vi "运维调试_总磷总氮.vi"() -> ()   [LabVIEW 2016, in "斯坦道仪器.lvlib"]
uses:
  <vilib>/Platform/TimedLoop/XDataNode/timing_clust.ctl
  <vilib>/Platform/TimedLoop/XDataNode/nitl_modes.ctl
  <vilib>/Platform/TimedLoop/XDataNode/wakeup.ctl
  <vilib>/Utility/miscctls.llb/LVPointTypeDef.ctl
  <vilib>/Utility/config.llb/Read Key (Double).vi
  <vilib>/Utility/config.llb/Write Key (Double).vi
  <vilib>/Platform/TimedLoop/XDataNode/XDataNode.xnode
  <vilib>/Platform/TimedLoop/XDataNode/XDNodeRunTimeDep.lvlib
  <vilib>/Utility/config.llb/NI_LVConfig.lvlib
panel:
  out "字符串":string
  out "总氮稀释倍数":dbl
  out "固件版本号":string
  in  "数组":string[](array[string])
  in  "备用系数写入":bool
  in  "备用系数读取":bool
  in  "备用系数":T1
  in  "量程切换阈值写入":bool
  in  "量程切换阈值读取":bool
  in  "量程切换阈值":cluster{"阈值":dbl, "标液浓度":dbl}
  in  "参数下拉列表":enum16{"总磷", "总氮"}(ring)
  in  "量程下拉列表":enum16{"低量程", "高量程"}(ring)
  in  "测量模式下拉列表":enum16{"水样测量", "空白核查", "跨度核查", "标样核查", "加标回收"}(ring)
  in  "公式":cluster{"X^2":dbl, "X":dbl, "b":dbl}
  in  "写公式":bool
  in  "读公式":bool
  in  "精度":dbl=4.0
  in  "样品5 F0":dbl
  in  "样品5 F1":dbl
  in  "样品4 F1":dbl
  in  "样品4 F0":dbl
  in  "样品3 F0":dbl
  in  "样品3 F1":dbl
  in  "样品2 F0":dbl
  in  "样品2 F1":dbl
  in  "样品1 F1":dbl
  in  "样品1 F0":dbl
  in  "method":u16(ring) items=["最小二乘", "最小绝对残差", "Bisquare"]
  in  "模型":enum32{"线性", "多项式"}(ring)
  out "r^2":dbl format="%.7g"
  out "拟合公式":string
  in  "样品2启用":bool
  in  "样品5启用":bool
  in  "样品4启用":bool
  in  "样品3启用":bool
  in  "样品1启用":bool
  in  "标液浓度5":dbl
  out "测量吸光度5":dbl
  in  "标液浓度4":dbl
  out "测量吸光度4":dbl
  in  "标液浓度3":dbl
  out "测量吸光度3":dbl
  in  "标液浓度2":dbl
  out "测量吸光度2":dbl
  out "测量吸光度1":dbl
  in  "标液浓度1":dbl
  out "XY图":cluster{"X Values":dbl[], "Y Values":dbl[]}[](graph)
  in  "返回":bool
  in  "设置":bool
  out "序列号":string="序列号"
  out "总氮测量数据":T2(xcontrol)
  out "总磷测量数据":T2(xcontrol)
  out "集成报警信息":string
  out "设置值":dbl
  out "定时启动":bool
  out "总磷总氮运行状态":T3(xcontrol)
  in  "停止":bool
  in  "手动启动":bool
  in  "单步测试":bool
  in  "总磷氨氮调试":u16[](xcontrol)
  out "F3":sgl format="%#.6f"
  out "F2":sgl format="%#.6f"
  out "F1":sgl format="%#.6f"
  out "F0":sgl format="%#.6f"
  out "多列列表框":i32(listbox)
  # "COM5"
  # "参数设置"
  # "标液浓度"
  # "F0"
  # "F1"
  # "吸光值显示"
  # "样品一"
  # "辅\n助\n计\n算\n区"
  # "样品二"
  # "样品三"
  # "样品四"
  # "样品五"
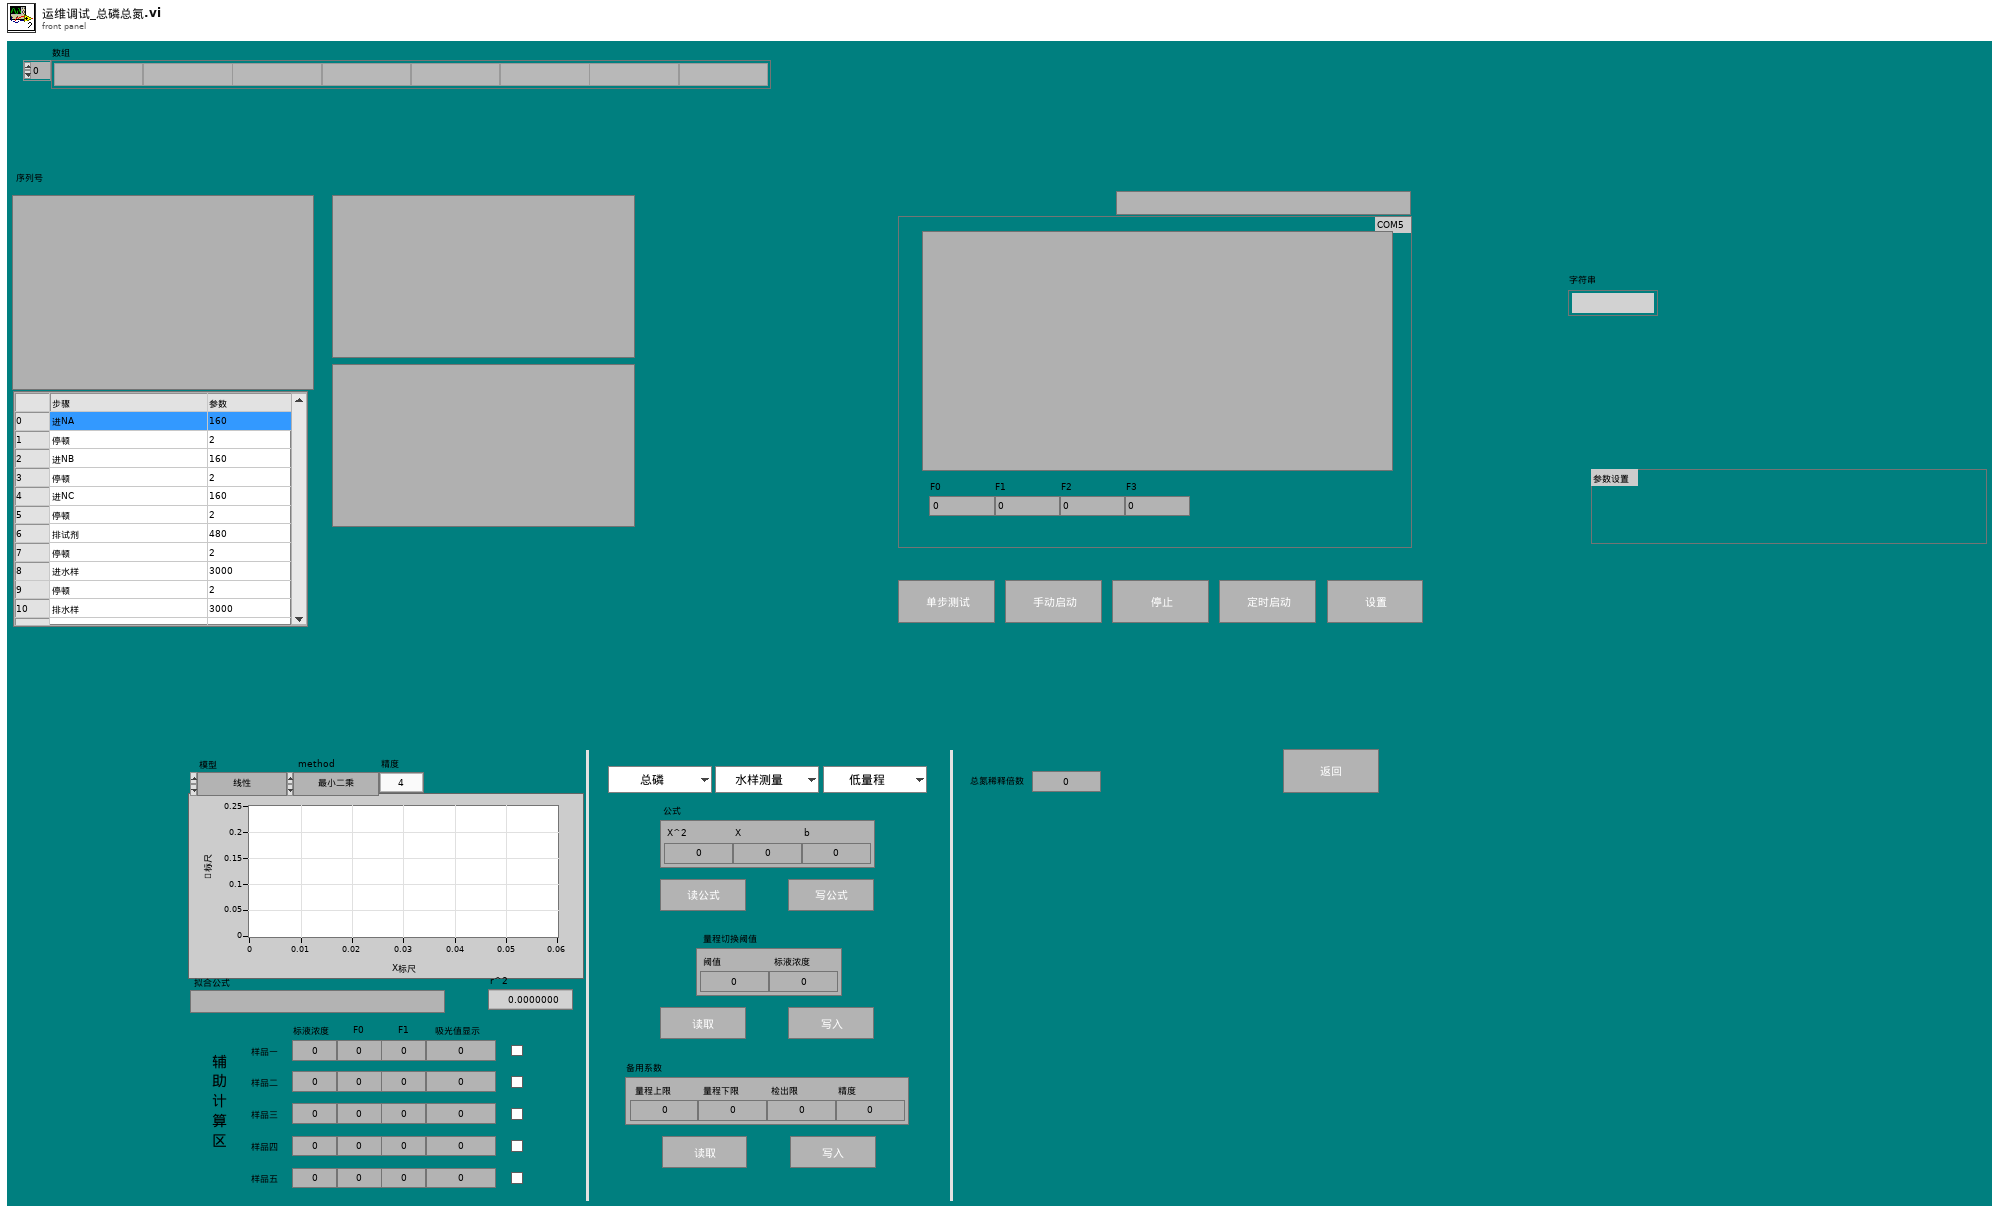
[diagram p1: front panel]
types:
  T1 = cluster{"量程上限":dbl, "量程下限":dbl, "检出限":dbl, "精度":dbl}
  T2 = cluster{"flowid":u16, "测量精度":u16, "测量数据区":cluster{"因子编码":u32, "单位":u16, "标样参考值":sgl, "水样数据时间":timestamp, "水样实测值":sgl, "水样数据标识":string, "标样数据时间":timestamp, "标样实测值":sgl, "标样数据标识":string, "空白数据时间":timestamp, "空白实测值":sgl, "空白数据标识":string, "零点核查数据时间":timestamp, "零点核查实测值":sgl, "零点核查数据标识":string, "跨度核查数据时间":timestamp, "跨度核查实测值":sgl, "跨度核查数据标识":string, "加标回收数据时间":timestamp, "加标回收实测值":sgl, "加标回收数据标识":string, "平行样数据时间":timestamp, "平行样实测值":sgl, "平行样数据标识":string, "F0":sgl, "F1":sgl, "F2":sgl, "F3":sgl, "F4":sgl, "F5":sgl, "F6":sgl, "F7":sgl, "温度":sgl, "湿度":sgl, "X值":sgl}}
  T3 = cluster{"系统时间":timestamp, "工作状态":enum16{"空闲", "水样测试", "标样核查", "零点核查", "跨度核查", "空白测试", "平行样测试", "加标回收", "空白校准", "标样校准", "初始化（清洗）"}, "测量模式":enum16{"待机", "连续模式", "周期模式", "定点模式", "受控模式", "手动模式"}, "告警代码":enum16{"无告警", "缺试剂告警", "缺水样告警", "缺蒸馏水告警", "缺标液告警", "仪表漏液告警", "标定异常告警", "超量程告警", "加热异常", "低试剂预警", "超上限告警", "超下限告警", "仪表内部其他异常", "滴定异常告警", "电极异常告警", "量程切换告警", "参数设置告警", "PH电极电位异常", "电导率电极异常", "浊度光度异常", "溶解氧电极异常", "溶解氧光强异常", "温度异常告警", "PH异常告警", "溶解氧异常告警", "电导率异常告警", "浊度异常告警", "叶绿素异常告警", "藻密度异常告警", "蓝绿藻异常告警", "ORP异常告警", "氨氮异常告警", "清洁刷异常告警", "SD卡异常告警", "蓝牙异常告警", "Wifi异常告警", "流程异常告警"}, "故障代码":enum16{"无故障", "电机故障", "温度故障", "通讯故障", "滴定故障"}, "日志代码":u16, "软件版本":u16, "F0":sgl, "F1":sgl, "F2":sgl, "F3":sgl, "T":sgl, "H":sgl, "id":u16, "flowid":u16, "量程":u16}
  T4 = enum16{"待机", "启动氨氮", "氨氮测量中", "启动总磷", "总磷测量中", "延时"}
  T5 = typedef "LVPointTypeDef.ctl" = cluster{"Horizontal":i16, "Vertical":i16}
  T6 = cluster{"因子编码":u32, "单位":u16, "标样参考值":sgl, "水样数据时间":timestamp, "水样实测值":sgl, "水样数据标识":string, "标样数据时间":timestamp, "标样实测值":sgl, "标样数据标识":string, "空白数据时间":timestamp, "空白实测值":sgl, "空白数据标识":string, "零点核查数据时间":timestamp, "零点核查实测值":sgl, "零点核查数据标识":string, "跨度核查数据时间":timestamp, "跨度核查实测值":sgl, "跨度核查数据标识":string, "加标回收数据时间":timestamp, "加标回收实测值":sgl, "加标回收数据标识":string, "平行样数据时间":timestamp, "平行样实测值":sgl, "平行样数据标识":string, "F0":sgl, "F1":sgl, "F2":sgl, "F3":sgl, "F4":sgl, "F5":sgl, "F6":sgl, "F7":sgl, "温度":sgl, "湿度":sgl, "X值":sgl}
  T7 = enum16{"空闲", "水样测试", "标样核查", "零点核查", "跨度核查", "空白测试", "平行样测试", "加标回收", "空白校准", "标样校准", "初始化（清洗）"}
  T8 = typedef "XDNodeRunTimeDep.lvlib/timing_clust.ctl" = cluster{"Expected End [f-1]":u64, "Actual End [f-1]":u64, "Finished Late? [f-1]":bool, "Expected End [i-1]":u64, "Actual End [i-1]":u64, "Finished Late? [i-1]":bool, "Expected Start [i]":u64, "Actual Start [i]":u64, "Expected Start [f]":u64, "Actual Start [f]":u64, "Source Name":string, "Structure Name":string, "Period":i64, "Deadline":i64, "Offset":i64, "Start":i64, "Priority":i32, "Timeout":i32, "Mode":T9, "Wakeup Reason":T10, "Error":errorcluster, "Source Type":string, "Secondary Source Type":string, "Global End Time":u64, "Global Start Time":u64, "Frame Duration":u64, "Iteration Duration":u64, "Assigned CPU":i32, "I/O Scan Engine Mode":u32}
  T9 = typedef "XDNodeRunTimeDep.lvlib/nitl_modes.ctl" = enum32{"No Change", "Process missed periods, maintain original phase", "Discard missed periods, maintain original phase", "Process missed periods, ignore original phase", "Discard missed periods, ignore original phase"}
  T10 = typedef "XDNodeRunTimeDep.lvlib/wakeup.ctl" = enum32{"Normal", "Aborted", "Asynchronous wakeup", "Timing source error", "Timed loop error", "Timeout"}
  T11 = cluster{"启动模式":enum16{"标液测量", "水样测量", "零液测量", "盲样测量", "加标回收"}, "启动参数":u16, "量程":enum16{"低量程", "高量程"}}
  T12 = cluster{"时间标识":timestamp, "设备":string, "日志信息":string, "流程参数":string}
  T13 = cluster{"时间标识":timestamp, "设备":string, "日志信息":string}
  T14 = enum16{"无告警", "缺试剂告警", "缺水样告警", "缺蒸馏水告警", "缺标液告警", "仪表漏液告警", "标定异常告警", "超量程告警", "加热异常", "低试剂预警", "超上限告警", "超下限告警", "仪表内部其他异常", "滴定异常告警", "电极异常告警", "量程切换告警", "参数设置告警", "PH电极电位异常", "电导率电极异常", "浊度光度异常", "溶解氧电极异常", "溶解氧光强异常", "温度异常告警", "PH异常告警", "溶解氧异常告警", "电导率异常告警", "浊度异常告警", "叶绿素异常告警", "藻密度异常告警", "蓝绿藻异常告警", "ORP异常告警", "氨氮异常告警", "清洁刷异常告警", "SD卡异常告警", "蓝牙异常告警", "Wifi异常告警", "流程异常告警"}
  T15 = typedef "LVRowAndColumnUnsignedTypeDef.ctl" = cluster{"Row":u32, "Column":u32}
  T16 = typedef "NI_LVConfig.lvlib/Config Data RefNum.ctl" = refnum<k1>
  T17 = cluster{"站号":u16, "量程切换":enum32{"H", "L", "AUTO"}, "控制命令":enum16{"启动测量", "标样核查", "零点核查", "跨度核查", "空白测试", "平行样测试", "加标回收", "空白校准", "标样校准", "初始化（清洗）", "停止测试", "仪器重启", "校时", "模式设置", "测量间隔设置", "盲样测试"}, "模式设置":enum16{"待机", "连续模式", "周期模式", "定点模式", "受控模式", "手动模式"}, "测量间隔":u16}
  T18 = cluster{"站号":u16, "量程切换":enum32{"H", "L", "AUTO"}, "控制命令":enum16{"启动测量", "标样核查", "零点核查", "跨度核查", "空白测试", "平行样测试", "加标回收", "空白校准", "标样校准", "初始化（清洗）", "停止测试", "仪器重启", "校时", "模式设置", "测量间隔设置"}, "模式设置":enum16{"待机", "连续模式", "周期模式", "定点模式", "受控模式", "手动模式"}, "测量间隔":u16}
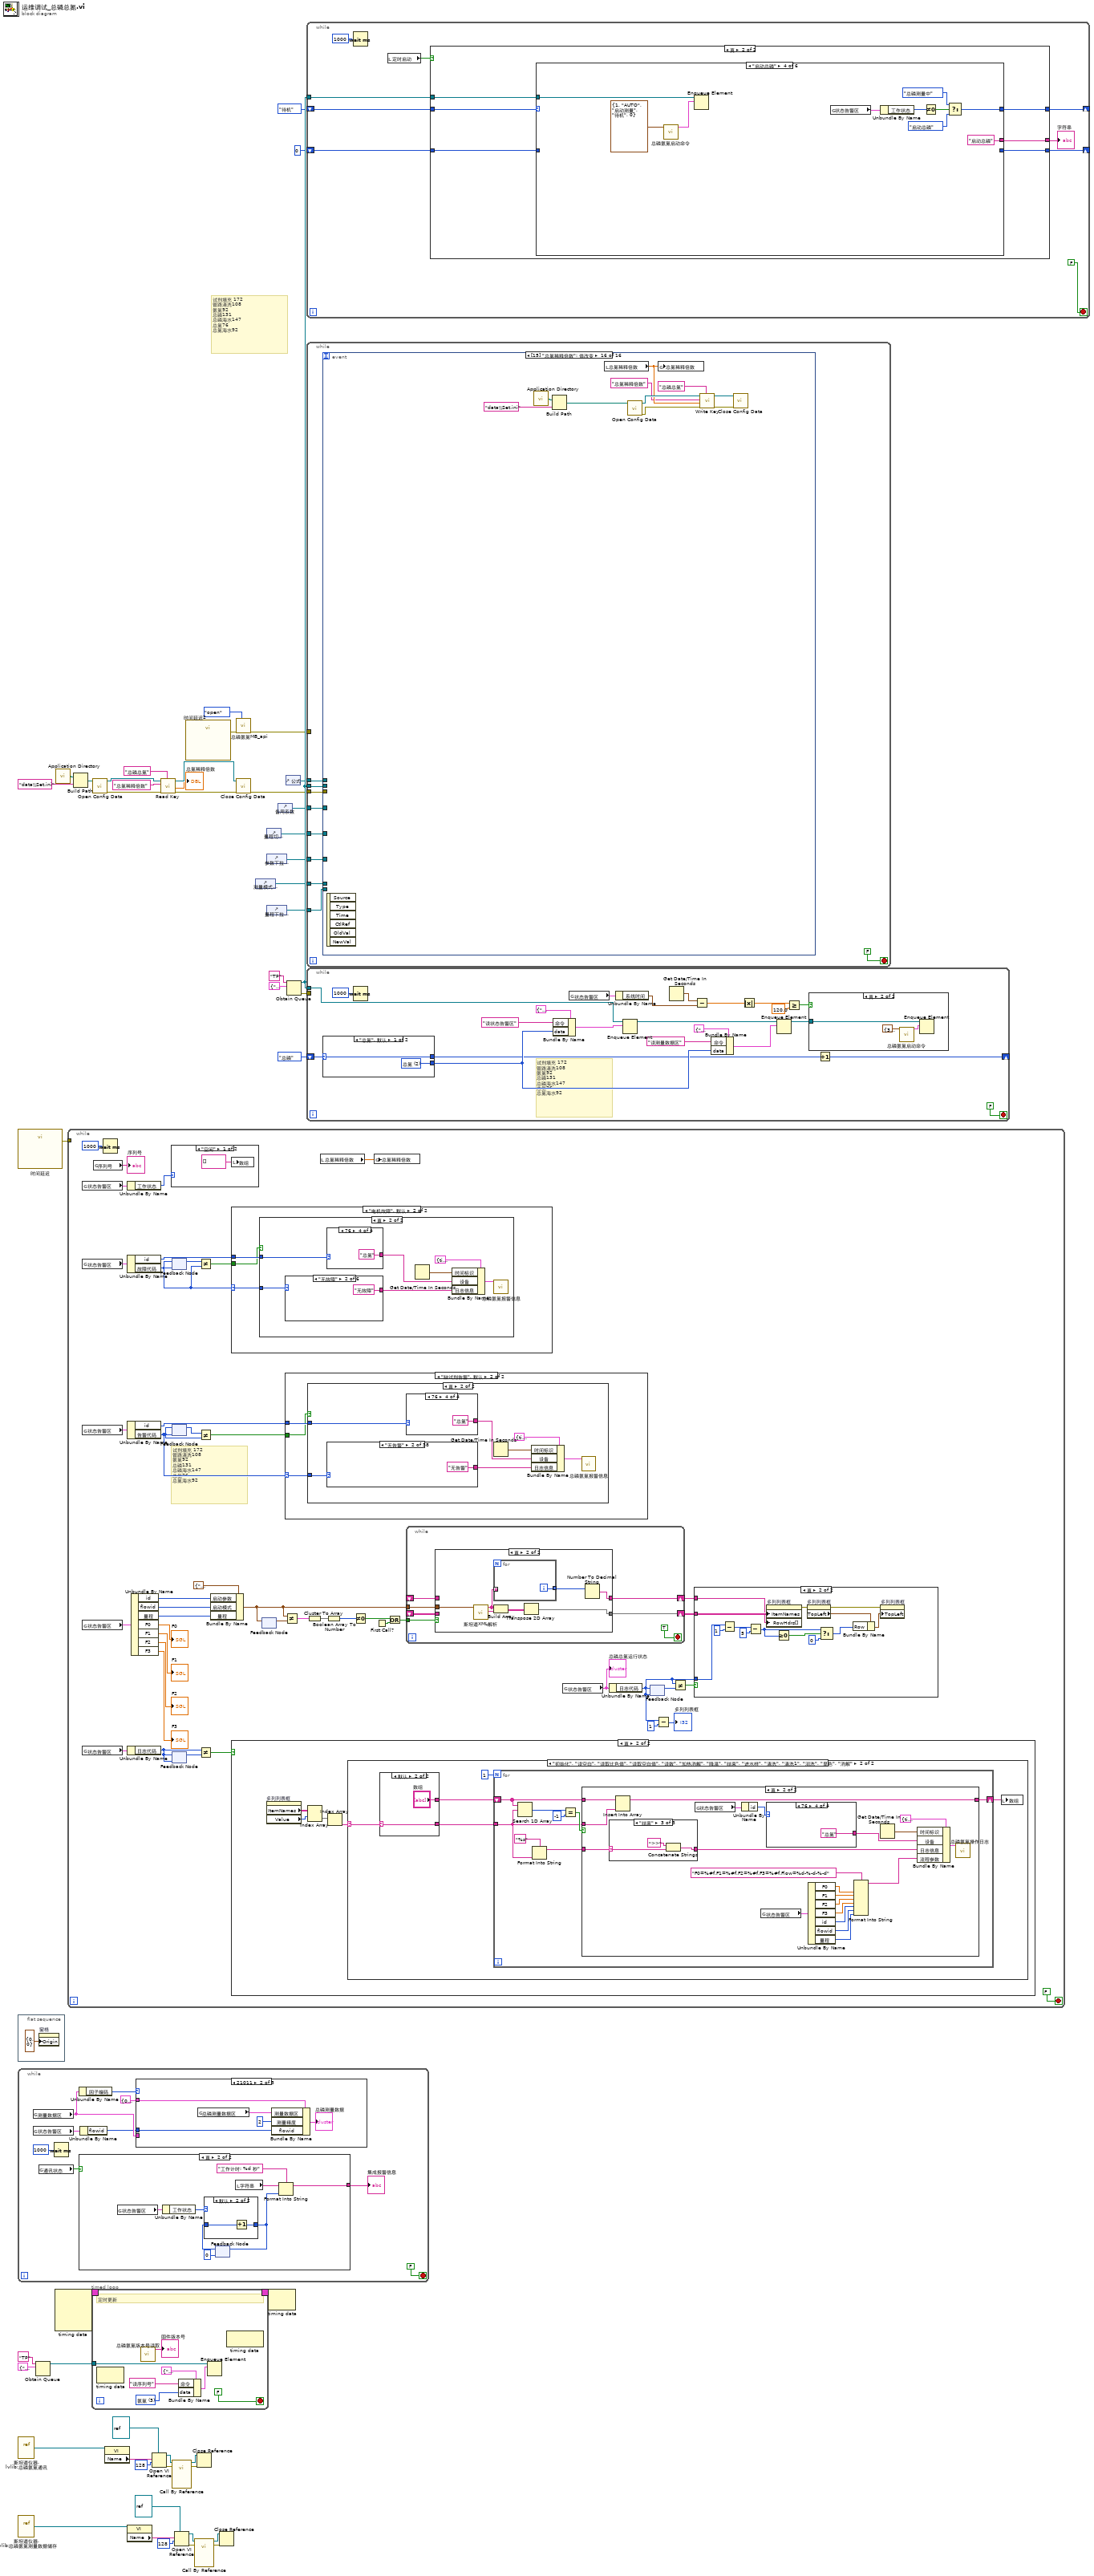
[diagram p0: block diagram]
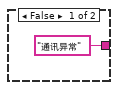
[diagram p2: hidden frame]
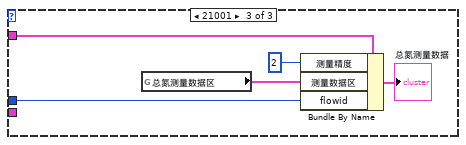
[diagram p5: hidden frame]
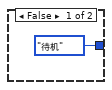
[diagram p6: hidden frame]
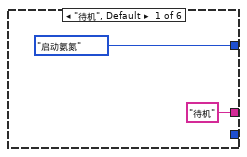
[diagram p7: hidden frame]
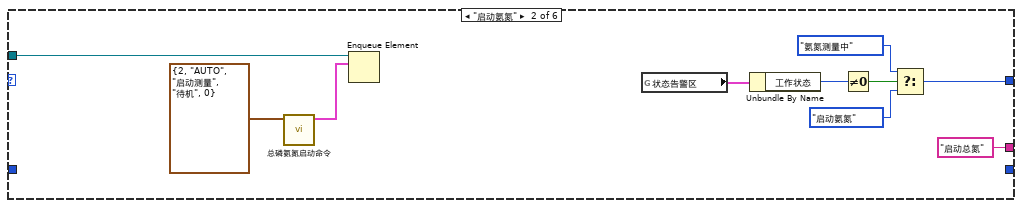
[diagram p8: hidden frame]
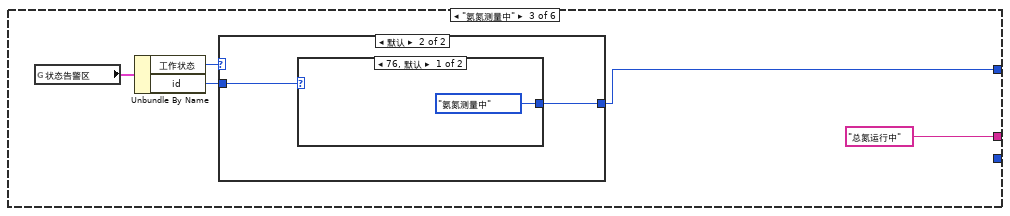
[diagram p9: hidden frame]
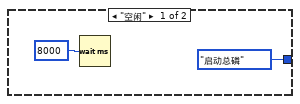
[diagram p10: hidden frame]
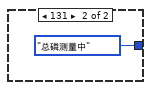
[diagram p11: hidden frame]
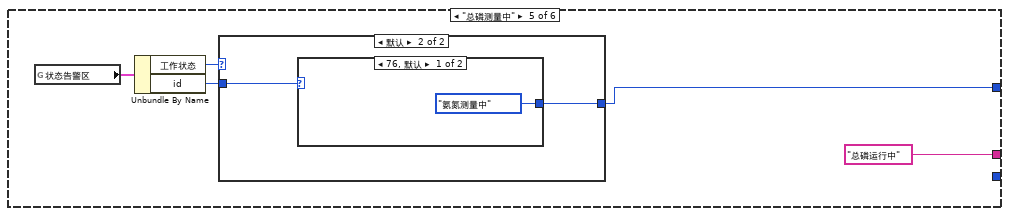
[diagram p12: hidden frame]
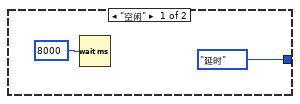
[diagram p13: hidden frame]
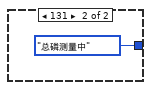
[diagram p14: hidden frame]
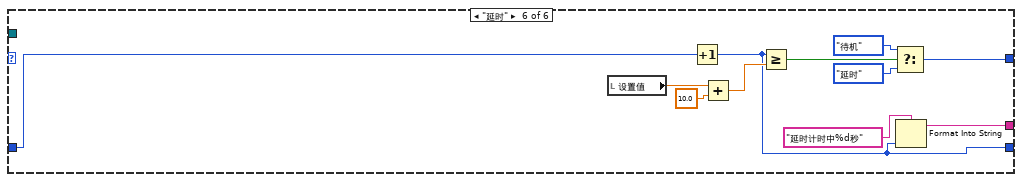
[diagram p15: hidden frame]
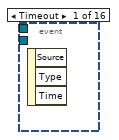
[diagram p16: hidden frame]
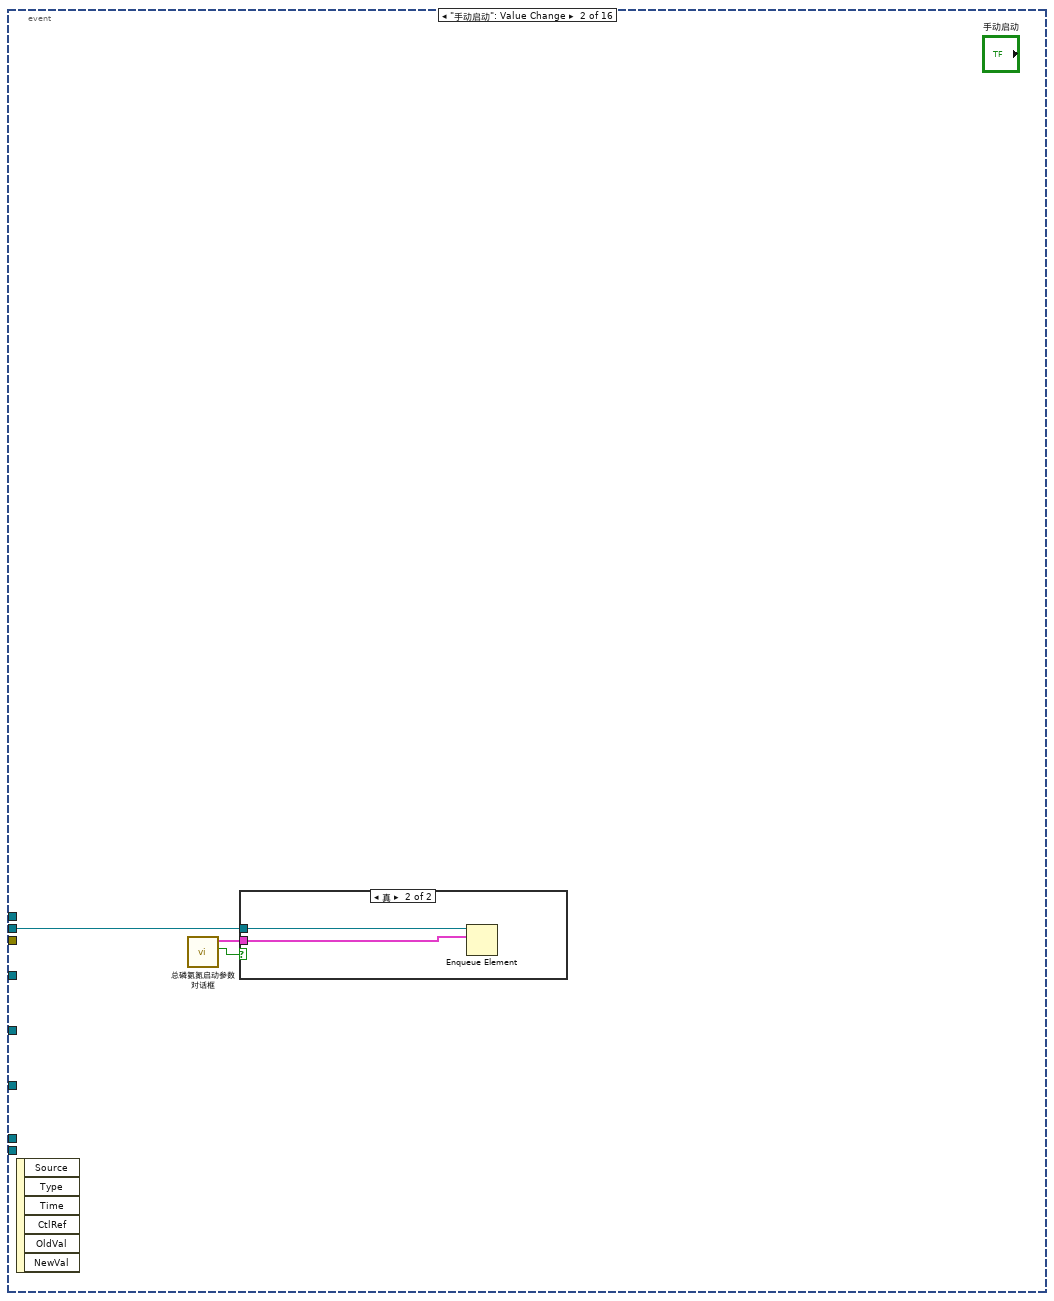
[diagram p17: hidden frame]
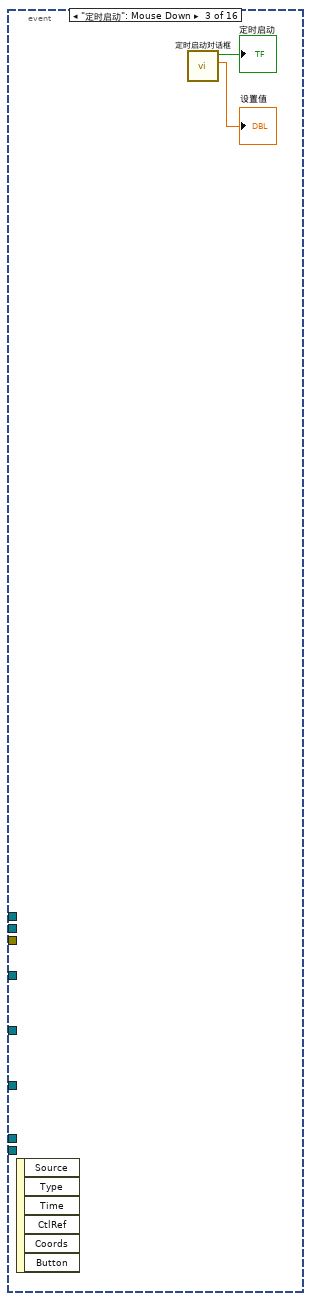
[diagram p19: hidden frame]
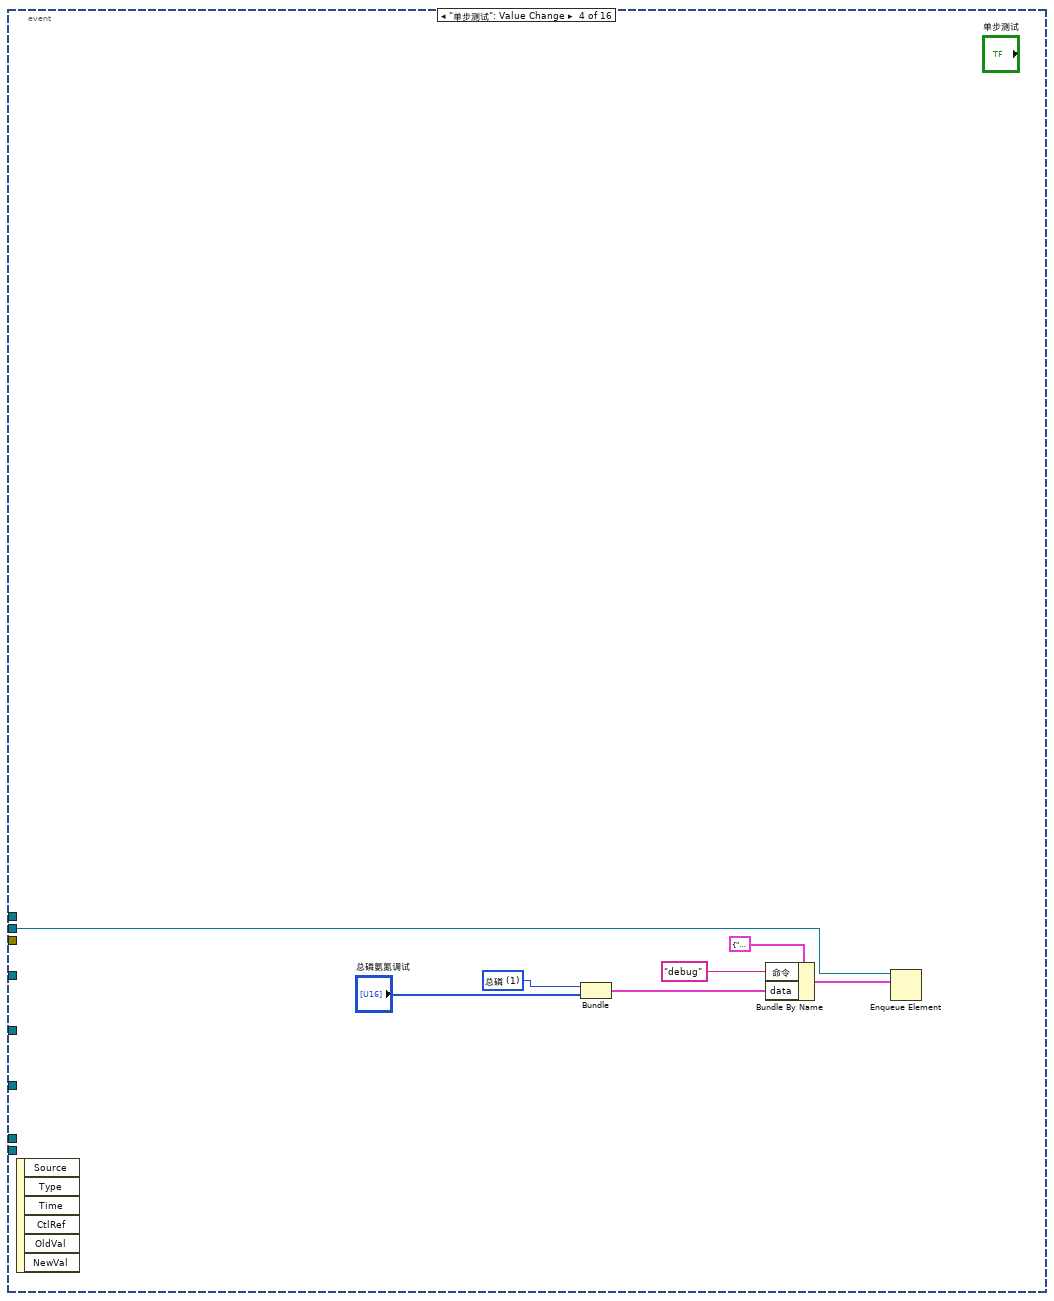
[diagram p20: hidden frame]
diagram:
  # "试剂填充 172 \n管路清洗108\n氨氮92\n总磷131\n总磷海水147\n总氮76\n总氮海水92"
  n1 = call "时间延迟"() -> ("error out"=w20:errorcluster)  [unwired: 11 in]
  n2 = flat-sequence {
    frame #0 {
      n3 = property on="窗格" class="Pane"("Origin"=T5 {"Horizontal"=0, "Vertical"=0} ("原点")) -> ()  [unwired: 2 in, 2 out]
    }
  }
  n4 = while {
    stop <- FALSE stop-if-true
    n5 = global read "VAR总磷氨氮全局变量.vi" "测量数据区"() -> (w57:T6)
    n6 = global read "VAR总磷氨氮全局变量.vi" "状态告警区"() -> (w53:T3)
    n7 = global read "VAR总磷氨氮全局变量.vi" "通讯状态"() -> (w55:bool)
    n8 = Wait (ms)(milliseconds to wait=u32 1000 ("等待时间（毫秒）")) -> ()  [unwired: 1 out]
    n9 = Unbundle By Name(w57) -> ("因子编码"=w56:u32)
    n10 = case shown="真" w55 {
      tunnel: ["通讯异常" ("集成报警信息") w62] -> w54
      frame False {
      }
      frame True {
        n11 = global read "VAR总磷氨氮全局变量.vi" "状态告警区"() -> (w68:T3)
        n12 = Unbundle By Name(w68) -> ("工作状态"=w67:T7)
        n13 = feedback #1(0) -> (w65:i32)
        n14 = case shown="默认" w67 {
          tunnel: w65 -> [_ w70]
          tunnel: [_ w69] -> w63
          frame "空闲" {
          }
          frame Default {
            n15 = Increment(x=w70) -> (x+1=w69:i32)
          }
        }
        n16 = feedback-in #1(w63) -> ()
        n17 = local read "字符串"() -> (w61:string)
        n18 = Format Into String(format string="工作计时: %d 秒" ("格式字符串"), initial string=w61, w63) -> (resulting string=w62:string)  [unwired: 1 in, 1 out]
      }
    }
    "集成报警信息" <- w54
    n19 = Unbundle By Name(w53) -> ("flowid"=w52:u16)
    n20 = case shown="21011" w56 {
      tunnel: w57 -> [_ _ _]
      tunnel: w52 -> [_ w73 w79]
      tunnel: T2 {"flowid"=0, "测量精度"=0, "测量数据区"={"因子编码"=0, "单位"=0, "标样参考值"=0.0, "水样数据时间"=timestamp(0 s since 1904-01-01), "水样实测值"=0.0, "水样数据标识"="", "标样数据时间"=timestamp(0 s since 1904-01-01), "标样实测值"=0.0, "标样数据标识"="", "空白数据时间"=timestamp(0 s since 1904-01-01), "空白实测值"=0.0, "空白数据标识"="", "零点核查数据时间"=timestamp(0 s since 1904-01-01), "零点核查实测值"=0.0, "零点核查数据标识"="", "跨度核查数据时间"=timestamp(0 s since 1904-01-01), "跨度核查实测值"=0.0, "跨度核查数据标识"="", "加标回收数据时间"=timestamp(0 s since 1904-01-01), "加标回收实测值"=0.0, "加标回收数据标识"="", "平行样数据时间"=timestamp(0 s since 1904-01-01), "平行样实测值"=0.0, "平行样数据标识"="", "F0"=0.0, "F1"=0.0, "F2"=0.0, "F3"=0.0, "F4"=0.0, "F5"=0.0, "F6"=0.0, "F7"=0.0, "温度"=0.0, "湿度"=0.0, "X值"=0.0}} ("总氮测量数据") -> [_ w72 w78]
      frame Default {
      }
      frame 21011 {
        n21 = global read "VAR总磷氨氮全局变量.vi" "总磷测量数据区"() -> (w71:T6)
        n22 = Bundle By Name(cluster=w72, "测量数据区"=w71, "测量精度"=u16 2, "flowid"=w73) -> (→"总磷测量数据":T2)
      }
      frame 21001 {
        n23 = global read "VAR总磷氨氮全局变量.vi" "总氮测量数据区"() -> (w76:T6)
        n24 = Bundle By Name(cluster=w78, "测量精度"=u16 2, "测量数据区"=w76, "flowid"=w79) -> (→"总氮测量数据":T2)
      }
    }
  }
  n25 = vi-ref "斯坦道仪器.lvlib:总磷氨氮通讯.vi"() -> (w43:refnum<vi>)
  n26 = vi-ref "斯坦道仪器.lvlib:总磷氨氮测量数据储存.vi"() -> (w35:refnum<vi>)
  n27 = Obtain Queue(name (unnamed)="TP" ("名称（未命名）"), element data type=cluster{"命令":string, "data":variant} {"命令"="", "data"=variant}) -> (queue out=w13:refnum<queue>)  [unwired: 3 in, 2 out]
  n28 = node-c288() -> (w17:T8)  [unwired: 4 in]
  n29 = call <vilib>:"Application Directory.vi"() -> ("Application Directory"=w7:path)
  n30 = while {
    tunnel: w20 -> [_]
    stop <- FALSE stop-if-true
    # "试剂填充 172 \n管路清洗108\n氨氮92\n总磷131\n总磷海水147\n总氮76\n总氮海水92"
    n31 = global read "VAR总磷氨氮全局变量.vi" "状态告警区"() -> (w90:T3)
    n32 = global read "VAR总磷氨氮全局变量.vi" "状态告警区"() -> (w95:T3)
    n33 = global read "VAR总磷氨氮全局变量.vi" "状态告警区"() -> (w100:T3)
    n34 = global read "VAR总磷氨氮全局变量.vi" "状态告警区"() -> (w112:T3)
    n35 = global read "VAR总磷氨氮全局变量.vi" "状态告警区"() -> (w87:T3)
    n36 = global read "VAR总磷氨氮全局变量.vi" "序列号"() -> (→"序列号":string)
    n37 = Wait (ms)(milliseconds to wait=u32 1000 ("等待时间（毫秒）")) -> ()  [unwired: 1 out]
    n38 = Unbundle By Name(w90) -> ("工作状态"=w89:T7)
    n39 = Unbundle By Name(w95) -> ("id"=w94:u16, "故障代码"=w91:enum16{"无故障", "电机故障", "温度故障", "通讯故障", "滴定故障"})
    n40 = Unbundle By Name(w100) -> ("id"=w99:u16, "告警代码"=w96:T14)
    n41 = Unbundle By Name(w87) -> ("日志代码"=w86:u16)
    n42 = Unbundle By Name(w112) -> ("id"=w109:u16, "flowid"=w111:u16, "量程"=w110:u16, "F0"=→"F0":sgl, "F1"=→"F1":sgl, "F2"=→"F2":sgl, "F3"=→"F3":sgl)
    n43 = case shown="\"空闲\"" w89 {
      frame "空闲" {
        n44 = local write "数组"(string[] [] ("数组")) -> ()
      }
      frame "水样测试", Default {
      }
    }
    n45 = feedback #2(w91) -> (w92:enum16{"无故障", "电机故障", "温度故障", "通讯故障", "滴定故障"})
    n46 = feedback-in #2(w91) -> ()
    n47 = feedback #3(w96) -> (w97:T14)
    n48 = feedback-in #3(w96) -> ()
    n49 = feedback #4(w86) -> (w88:u16)
    n50 = feedback-in #4(w86) -> ()
    n51 = Not Equal?(x=w92, y=w91) -> (x != y?=w93:bool)
    n52 = Not Equal?(x=w97, y=w96) -> (x != y?=w98:bool)
    n53 = Not Equal?(x=w86, y=w88) -> (x != y?=w85:bool)
    n54 = Bundle By Name(cluster=T11 {"启动模式"=enum."加标回收", "启动参数"=1, "量程"=enum."低量程"} ("参数簇"), "启动参数"=w109, "启动模式"=w111, "量程"=w110) -> (w102:T11)
    n55 = case shown="\"电机故障\", 默认" w91 {
      selector: w91 -> [_ w181]
      tunnel: w94 -> [_ w182]
      tunnel: w93 -> [_ w180]
      frame "无故障" {
      }
      frame "电机故障", Default {
        n56 = case shown="真" w180 {
          tunnel: w182 -> [_ w189]
          tunnel: w181 -> [_ w184]
          frame False {
          }
          frame True {
            n57 = case shown="\"无故障\"" w184 {
              selector: w184 -> [w191 _ _ _ _ _]
              tunnel: [w190 "无故障" "电机故障" "温度故障" "通讯故障" "滴定故障"] -> w183
              frame Default {
                n58 = Format Into String(format string="%d" ("格式字符串"), initial string="未知" ("工作状态"), w191) -> (resulting string=w190:string)  [unwired: 1 in, 1 out]
              }
              frame "无故障" {
              }
              frame "电机故障" {
              }
              frame "温度故障" {
              }
              frame "通讯故障" {
              }
              frame "滴定故障" {
              }
            }
            n59 = case shown="76" w189 {
              tunnel: [_ "总磷" ("table输入") "氨氮" ("table输入") "总氮" ("table输入")] -> w185
              frame Default {
              }
              frame 131 {
              }
              frame 92 {
              }
              frame 76 {
              }
            }
            n60 = Get Date/Time In Seconds() -> (seconds since 1Jan1904=w186:timestamp)
            n61 = Bundle By Name(cluster=T13 {"时间标识"=timestamp(0 s since 1904-01-01), "设备"="", "日志信息"=""} ("data in"), "时间标识"=w186, "设备"=w185, "日志信息"=w183) -> (w187:T13)
            n62 = call "总磷氨氮报警信息.vi"("data in"=w187) -> ()  [unwired: 11 in]
          }
        }
      }
    }
    n63 = case shown="真" w85 {
      frame False {
      }
      frame True {
        n64 = property on="多列列表框" class="MCListbox (严格)"() -> ("ItemNames"=w129:string[][], "Value"=w130:i32)  [unwired: 2 in, 2 out]
        n65 = Index Array(array=w129, index (row)=w130) -> (element=w128:string[])  [unwired: 1 in]
        n66 = Index Array(array=w128) -> (element=w127:string)  [unwired: 1 in]
        n67 = case shown="\"初始化\", \"读空白\", \"读取比色值\", \"读取空白值\", \"读数\", \"加热消解\", \"降温\", \"结束\", \"进水样\", \"清洗\", \"清洗1\", \"润洗\", \"显色\", \"消解\"" w127 {
          selector: w127 -> [_ w133]
          frame Default {
          }
          frame "初始化", "读空白", "读取比色值", "读取空白值", "读数", "加热消解", "降温", "结束", "进水样", "清洗", "清洗1", "润洗", "显色", "消解" {
            n68 = case shown="默认" w133 {
              selector: w133 -> [w137 w139]
              tunnel: [w137 w139] -> w132
              tunnel: [string[] [] ("数组") "数组"] -> w131
              frame "读数" {
              }
              frame Default {
              }
            }
            n69 = for {
              N: 1 -> [_]
              tunnel: w132 -> [w141]
              shift-right: [w140] -> w134
              shift-left: w131 -> [w142]
              n70 = Search 1D Array(1D array=w142, element=w141) -> (index of element=w145:i32)  [unwired: 1 in]
              n71 = Format Into String(format string="%s" ("格式字符串"), w141) -> (resulting string=w146:string)  [unwired: 2 in, 1 out]
              n72 = Equal?(x=w145, y=-1) -> (x = y?=w143:bool)
              n73 = case shown="真" w143 {
                tunnel: w146 -> [_ w150]
                tunnel: w142 -> [w148 w154]
                tunnel: w141 -> [_ w153]
                tunnel: [w148 w152] -> w140
                frame False {
                }
                frame True {
                  n74 = case shown="\"结束\"" w150 {
                    selector: w150 -> [w170 w173 w176]
                    tunnel: [w170 w172 w175] -> w149
                    frame Default {
                    }
                    frame "初始化" {
                      n75 = Concatenate Strings("<<" ("字符串"), w173) -> (w172:string)
                    }
                    frame "结束" {
                      n76 = Concatenate Strings(">>" ("字符串"), w176) -> (w175:string)
                    }
                  }
                  n77 = Insert Into Array(array=w154, new element=w153) -> (w152:string[])  [unwired: 1 in]
                  n78 = global read "VAR总磷氨氮全局变量.vi" "状态告警区"() -> (w169:T3)
                  n79 = Unbundle By Name(w169) -> ("id"=w168:u16)
                  n80 = global read "VAR总磷氨氮全局变量.vi" "状态告警区"() -> (w164:T3)
                  n81 = case shown="76" w168 {
                    tunnel: [_ "总磷" ("table输入") "氨氮" ("table输入") "总氮" ("table输入")] -> w166
                    frame Default {
                    }
                    frame 131 {
                    }
                    frame 92 {
                    }
                    frame 76 {
                    }
                  }
                  n82 = Unbundle By Name(w164) -> ("F0"=w161:sgl, "F1"=w160:sgl, "F2"=w159:sgl, "F3"=w158:sgl, "id"=w157:u16, "flowid"=w156:u16, "量程"=w155:u16)
                  n83 = Format Into String(format string="F0=%#f,F1=%#f,F2=%#f,F3=%#f,Flow=%d-%-d-%-d" ("格式字符串"), w161, w160, w159, w158, w157, w156, w155) -> (resulting string=w162:string)  [unwired: 2 in, 1 out]
                  n84 = Get Date/Time In Seconds() -> (seconds since 1Jan1904=w165:timestamp)
                  n85 = Bundle By Name(cluster=T12 {"时间标识"=timestamp(0 s since 1904-01-01), "设备"="", "日志信息"="", "流程参数"=""} ("data in"), "时间标识"=w165, "设备"=w166, "日志信息"=w149, "流程参数"=w162) -> (w167:T12)
                  n86 = call "总磷氨氮操作日志.vi"("data in"=w167) -> ()  [unwired: 11 in]
                }
              }
            }
            n87 = local write "数组"(w134) -> ()
          }
        }
      }
    }
    n88 = feedback #5() -> (w118:T11)  [unwired: 1 in]
    n89 = feedback-in #5(w102) -> ()
    n90 = Not Equal?(x=w102, y=w118) -> (x != y?=w119:cluster{"启动模式":bool, "启动参数":bool, "量程":bool})
    n91 = case shown="\"缺试剂告警\", 默认" w96 {
      selector: w96 -> [_ w203]
      tunnel: w99 -> [_ w204]
      tunnel: w98 -> [_ w202]
      frame "无告警" {
      }
      frame "缺试剂告警", Default {
        n92 = case shown="真" w202 {
          tunnel: w204 -> [_ w211]
          tunnel: w203 -> [_ w205]
          frame False {
          }
          frame True {
            n93 = case shown="\"无告警\"" w205 {
              selector: w205 -> [w213 _ _ _ _ _ _ _ _ _ _ _ _ _ _ _ _ _ _ _ _ _ _ _ _ _ _ _ _ _ _ _ _ _ _ _ _ _]
              tunnel: [w212 "无告警" "缺试剂告警" "缺水样告警" "缺蒸馏水告警" "缺标液告警" "仪表漏液告警" "标定异常告警" "超量程告警" "加热异常" "低试剂预警" "超上限告警" "超下限告警" "仪表内部其他异常" "滴定异常告警" "电极异常告警" "量程切换告警" "参数设置告警" "PH电极电位异常" "电导率电极异常" "浊度光度异常" "溶解氧电极异常" "溶解氧光强异常" "温度异常告警" "PH异常告警" "溶解氧异常告警" "电导率异常告警" "浊度异常告警" "叶绿素异常告警" "藻密度异常告警" "蓝绿藻异常告警" "ORP异常告警" "氨氮异常告警" "清洁刷异常告警" "SD卡异常告警" "蓝牙异常告警" "WiFi异常告警" "流程异常告警"] -> w206
              frame Default {
                n94 = Format Into String(format string="%d" ("格式字符串"), initial string="未知" ("工作状态"), w213) -> (resulting string=w212:string)  [unwired: 1 in, 1 out]
              }
              frame "无告警" {
              }
              frame "缺试剂告警" {
              }
              frame "缺水样告警" {
              }
              frame "缺蒸馏水告警" {
              }
              frame "缺标液告警" {
              }
              frame "仪表漏液告警" {
              }
              frame "标定异常告警" {
              }
              frame "超量程告警" {
              }
              frame "加热异常" {
              }
              frame "低试剂预警" {
              }
              frame "超上限告警" {
              }
              frame "超下限告警" {
              }
              frame "仪表内部其他异常" {
              }
              frame "滴定异常告警" {
              }
              frame "电极异常告警" {
              }
              frame "量程切换告警" {
              }
              frame "参数设置告警" {
              }
              frame "PH电极电位异常" {
              }
              frame "电导率电极异常" {
              }
              frame "浊度光度异常" {
              }
              frame "溶解氧电极异常" {
              }
              frame "溶解氧光强异常" {
              }
              frame "温度异常告警" {
              }
              frame "PH异常告警" {
              }
              frame "溶解氧异常告警" {
              }
              frame "电导率异常告警" {
              }
              frame "浊度异常告警" {
              }
              frame "叶绿素异常告警" {
              }
              frame "藻密度异常告警" {
              }
              frame "蓝绿藻异常告警" {
              }
              frame "ORP异常告警" {
              }
              frame "氨氮异常告警" {
              }
              frame "清洁刷异常告警" {
              }
              frame "SD卡异常告警" {
              }
              frame "蓝牙异常告警" {
              }
              frame "Wifi异常告警" {
              }
              frame "流程异常告警" {
              }
            }
            n95 = case shown="76" w211 {
              tunnel: [_ "总磷" ("table输入") "氨氮" ("table输入") "总氮" ("table输入")] -> w207
              frame Default {
              }
              frame 131 {
              }
              frame 92 {
              }
              frame 76 {
              }
            }
            n96 = Get Date/Time In Seconds() -> (seconds since 1Jan1904=w208:timestamp)
            n97 = Bundle By Name(cluster=T13 {"时间标识"=timestamp(0 s since 1904-01-01), "设备"="", "日志信息"=""} ("data in"), "时间标识"=w208, "设备"=w207, "日志信息"=w206) -> (w209:T13)
            n98 = call "总磷氨氮报警信息.vi"("data in"=w209) -> ()  [unwired: 11 in]
          }
        }
      }
    }
    n99 = Cluster To Array(cluster=w119) -> (array=w120:bool[])
    n100 = local read "总氮稀释倍数"() -> (w81:dbl)
    n101 = Boolean Array To Number(Boolean array=w120) -> (number=w121:u32)
    n102 = Not Equal To 0?(x=w121) -> (x != 0?=w114:bool)
    n103 = global write "VAR总磷氨氮全局变量.vi" "总氮稀释倍数"(w81) -> ()
    n104 = First Call?() -> (First Call?: T/F=w115:bool)
    n105 = Or(x=w114, y=w115) -> (x .or. y?=w113:bool)
    n106 = while {
      tunnel: w113 -> [w262]
      tunnel: w102 -> [w261]
      shift-right: [w260] -> w117
      shift-left: _ -> [w256]
      shift-right: [w259] -> w116
      shift-left: _ -> [w257]
      stop <- TRUE stop-if-true
      n107 = case shown="真" w262 {
        tunnel: [w264 w271] -> w259
        tunnel: [w263 w270] -> w260
        tunnel: w261 -> [_ w265]
        tunnel: w257 -> [w264 _]
        tunnel: w256 -> [w263 _]
        frame False {
        }
        frame True {
          n108 = call "斯坦道XML解析.vi"("参数簇"=w265) -> ("步骤时间"=w266:string[], "步骤名"=w268:string[])  [unwired: 9 in]
          n109 = for {
            tunnel: w268 -> [_] mode=indexing
            tunnel: [w272] -> w269 mode=indexing
            i -> [w272]
          }
          n110 = Build Array(w268, w266) -> (w267:string[][])
          n111 = Transpose 2D Array(2D array=w267) -> (transposed array=w270:string[][])
          n112 = Number To Decimal String(number=w269) -> (decimal integer string=w271:string[])  [unwired: 1 in]
        }
      }
    }
    n113 = global read "VAR总磷氨氮全局变量.vi" "状态告警区"() -> (w103:T3)
    "总磷总氮运行状态" <- w103
    n114 = Unbundle By Name(w103) -> ("日志代码"=w83:u16)
    n115 = feedback-in #6(w83) -> ()
    n116 = feedback #6(w83) -> (w123:u16)
    n117 = Subtract(x=w83, y=1) -> (x-y=→"多列列表框":i32)
    n118 = Not Equal?(x=w83, y=w123) -> (x != y?=w122:bool)
    n119 = case shown="真" w122 {
      tunnel: w83 -> [_ w275]
      tunnel: w117 -> [_ w282]
      tunnel: w116 -> [_ w281]
      frame False {
      }
      frame True {
        n120 = Subtract(x=w275, y=1) -> (x-y=w273:i32)
        n121 = Subtract(x=w273, y=5) -> (x-y=w277:i32)
        n122 = property on="多列列表框" class="MCListbox (严格)"("ItemNames"=w282, "RowHdrs[]"=w281) -> (error out=w283:errorcluster)  [unwired: 2 in, 1 out]
        n123 = Greater Or Equal To 0?(x=w277) -> (x >= 0?=w276:bool)
        n124 = property on="多列列表框" class="MCListbox (严格)"(error in=w283) -> (error out=w284:errorcluster, "TopLeft"=w285:T15)  [unwired: 1 in, 1 out]
        n125 = Select(t=w277, s=w276, f=0) -> (s? t:f=w278:i32)
        n126 = Bundle By Name(cluster=w285, "Row"=w278) -> (w286:T15)
        n127 = property on="多列列表框" class="MCListbox (严格)"(error in=w284, "TopLeft"=w286) -> ()  [unwired: 1 in, 2 out]
      }
    }
  }
  n128 = Build Path(base path=w7, name or relative path="data\\Set.ini" ("名称或相对路径")) -> (appended path=w5:path)
  n129 = timed-loop {
    timing: w17 -> [_]
    timing-out: [_] -> w16
    tunnel: w13 -> [w289]
    stop <- FALSE stop-if-true
    w290 = u16 3 items=["总磷"=1, "氨氮"=3] ("站号")
    # "定时更新"
    n130 = node-c288() -> ()  [unwired: 1 in, 1 out]
    n131 = call "总磷氨氮版本号读取.vi"() -> ("固件版本号"=→"固件版本号":string)  [unwired: 11 in]
    n132 = Bundle By Name(cluster=cluster{"命令":string, "data":variant} {"命令"="", "data"=variant} ("元素"), "命令"="读序列号", "data"=w290) -> (w288:cluster{"命令":string, "data":variant})
    n133 = Enqueue Element(queue=w289, element=w288) -> ()  [unwired: 2 in, 3 out]
    n134 = node-c288() -> ()  [unwired: 1 in, 1 out]
  }
  n135 = call <vilib>:"Open Config Data.vi"("configuration file path"=w5) -> ("error out"=w9:errorcluster, "refnum"=w11:T16)  [unwired: 8 in, 1 out]
  n136 = property class="VI"(reference=w43) -> ("Name"=w42:string)  [unwired: 1 in, 2 out]
  n137 = property class="VI"(reference=w35) -> ("Name"=w28:string)  [unwired: 1 in, 2 out]
  n138 = Open VI Reference(type specifier VI Refnum (for type only)=refnum<vi> refnum, vi path=w42, options=128 ("选项")) -> (vi reference=w40:refnum<vi>, error out=w38:errorcluster)  [unwired: 3 in]
  n139 = call-poly <vilib>:"Read Key.vi"("section"="总磷总氮", "error in (no error)"=w9, "key"="总氮稀释倍数" ("section"), "refnum"=w11) -> ("error out"=w8:errorcluster, "value"=→"总氮稀释倍数":dbl, "refnum out"=w10:T16)  [unwired: 4 in, 1 out]
  n140 = call-by-ref "?"(reference=w40, error in=w38) -> (reference out=w36:refnum<vi>, error out=w37:errorcluster)  [unwired: 12 in]
  n141 = Open VI Reference(type specifier VI Refnum (for type only)=refnum<vi> refnum, vi path=w28, options=128 ("选项")) -> (vi reference=w30:refnum<vi>, error out=w32:errorcluster)  [unwired: 3 in]
  n142 = call "时间延迟2"() -> ("error out"=w12:errorcluster)  [unwired: 11 in]
  n143 = call-by-ref "?"(reference=w30, error in=w32) -> (reference out=w34:refnum<vi>, error out=w33:errorcluster)  [unwired: 12 in]
  n144 = Close Reference(reference=w36, error in (no error)=w37) -> ()  [unwired: 1 out]
  n145 = Close Reference(reference=w34, error in (no error)=w33) -> ()  [unwired: 1 out]
  n146 = call "总磷氨氮MB_api.vi"("STEP"=enum16{"open", "read", "write", "close"}."open", "Error in"=w12) -> ("error out"=w19:errorcluster)  [unwired: 7 in, 2 out]
  n147 = call <vilib>:"Close Config Data.vi"("error in (no error)"=w8, "refnum"=w10) -> ("error out"=w3:errorcluster)  [unwired: 8 in, 1 out]
  n148 = control-ref of="测量模式下拉列表"() -> (w24:refnum<vi>)
  n149 = control-ref of="量程切换阈值"() -> (w22:refnum<vi>)
  n150 = control-ref of="参数下拉列表"() -> (w25:refnum<vi>)
  n151 = control-ref of="量程下拉列表"() -> (w26:refnum<vi>)
  n152 = node-c288(w16) -> ()  [unwired: 1 out]
  n153 = control-ref of="备用系数"() -> (w21:refnum<vi>)
  n154 = control-ref of="公式"() -> (w23:refnum<vi>)
  n155 = Obtain Queue(name (unnamed)="TP" ("名称（未命名）"), element data type=cluster{"命令":string, "data":variant} {"命令"="", "data"=variant}) -> (queue out=w46:refnum<queue>, error out=w47:errorcluster)  [unwired: 3 in, 1 out]
  n156 = while {
    tunnel: w46 -> [w299]
    shift-right: [w300] -> _
    shift-left: T4."待机" -> [w301]
    shift-right: [w297] -> _
    shift-left: u32 0 ("等待时间（毫秒）") -> [w298]
    stop <- FALSE stop-if-true
    n157 = Wait (ms)(milliseconds to wait=u32 1000 ("等待时间（毫秒）")) -> ()  [unwired: 1 out]
    n158 = local read "定时启动"() -> (w302:bool)
    n159 = case shown="真" w302 {
      tunnel: w301 -> [_ w311]
      tunnel: [T4."待机" w310] -> w300
      tunnel: w299 -> [_ w309]
      tunnel: w298 -> [_ w308]
      tunnel: [_ w307] -> w297
      tunnel: [_ w306] -> w296
      frame False {
      }
      frame True {
        n160 = case shown="\"启动总磷\"" w311 {
          tunnel: [T4."启动氨氮" w318 w324 w338 w345 w364] -> w310
          tunnel: w309 -> [_ w323 _ w344 _ _]
          tunnel: w308 -> [_ _ _ _ _ w366]
          tunnel: [_ _ _ _ _ w358] -> w307
          tunnel: ["待机" ("字符串") "启动总氮" ("字符串") "总氮运行中" ("字符串") "启动总磷" ("字符串") "总磷运行中" ("字符串") w356] -> w306
          frame "待机", Default {
          }
          frame "启动氨氮" {
            n161 = call "总磷氨氮启动命令.vi"("参数"=T17 {"站号"=2, "量程切换"=enum."AUTO", "控制命令"=enum."启动测量", "模式设置"=enum."待机", "测量间隔"=0}) -> ("启动命令"=w316:cluster{"命令":string, "data":variant})  [unwired: 10 in]
            n162 = Enqueue Element(queue=w323, element=w316) -> ()  [unwired: 2 in, 3 out]
            n163 = global read "VAR总磷氨氮全局变量.vi" "状态告警区"() -> (w322:T3)
            n164 = Unbundle By Name(w322) -> ("工作状态"=w321:T7)
            n165 = Not Equal To 0?(x=w321) -> (x != 0?=w320:bool)
            n166 = Select(t=T4."氨氮测量中", s=w320, f=T4."启动氨氮") -> (s? t:f=w318:T4)
          }
          frame "氨氮测量中" {
            n167 = global read "VAR总磷氨氮全局变量.vi" "状态告警区"() -> (w327:T3)
            n168 = Unbundle By Name(w327) -> ("工作状态"=w325:T7, "id"=w326:u16)
            n169 = case shown="默认" w325 {
              tunnel: w326 -> [_ w332]
              tunnel: [T4."启动总磷" w331] -> w324
              frame "空闲" {
                n170 = Wait (ms)(milliseconds to wait=u32 8000 ("等待时间（毫秒）")) -> ()  [unwired: 1 out]
              }
              frame Default {
                n171 = case shown="76, 默认" w332 {
                  tunnel: [T4."氨氮测量中" T4."总磷测量中"] -> w331
                  frame 76, Default {
                  }
                  frame 131 {
                  }
                }
              }
            }
          }
          frame "启动总磷" {
            n172 = call "总磷氨氮启动命令.vi"("参数"=T17 {"站号"=1, "量程切换"=enum."AUTO", "控制命令"=enum."启动测量", "模式设置"=enum."待机", "测量间隔"=0}) -> ("启动命令"=w337:cluster{"命令":string, "data":variant})  [unwired: 10 in]
            n173 = Enqueue Element(queue=w344, element=w337) -> ()  [unwired: 2 in, 3 out]
            n174 = global read "VAR总磷氨氮全局变量.vi" "状态告警区"() -> (w339:T3)
            n175 = Unbundle By Name(w339) -> ("工作状态"=w340:T7)
            n176 = Not Equal To 0?(x=w340) -> (x != 0?=w341:bool)
            n177 = Select(t=T4."总磷测量中", s=w341, f=T4."启动总磷") -> (s? t:f=w338:T4)
          }
          frame "总磷测量中" {
            n178 = global read "VAR总磷氨氮全局变量.vi" "状态告警区"() -> (w348:T3)
            n179 = Unbundle By Name(w348) -> ("工作状态"=w346:T7, "id"=w347:u16)
            n180 = case shown="默认" w346 {
              tunnel: w347 -> [_ w353]
              tunnel: [T4."延时" w352] -> w345
              frame "空闲" {
                n181 = Wait (ms)(milliseconds to wait=u32 8000 ("等待时间（毫秒）")) -> ()  [unwired: 1 out]
              }
              frame Default {
                n182 = case shown="76, 默认" w353 {
                  tunnel: [T4."氨氮测量中" T4."总磷测量中"] -> w352
                  frame 76, Default {
                  }
                  frame 131 {
                  }
                }
              }
            }
          }
          frame "延时" {
            n183 = local read "设置值"() -> (w361:dbl)
            n184 = Increment(x=w366) -> (x+1=w358:u32)
            n185 = Add(x=w361, y=10.0) -> (x+y=w359:dbl)
            n186 = Greater Or Equal?(x=w358, y=w359) -> (x >= y?=w365:bool)
            n187 = Select(t=T4."待机", s=w365, f=T4."延时") -> (s? t:f=w364:T4)
            n188 = Format Into String(format string="延时计时中%d秒" ("格式字符串"), w358) -> (resulting string=w356:string)  [unwired: 2 in, 1 out]
          }
        }
      }
    }
    "字符串" <- w296
  }
  n189 = while {
    tunnel: w46 -> [w374]
    tunnel: w26 -> [w373]
    tunnel: w25 -> [w372]
    tunnel: w24 -> [w371]
    tunnel: w23 -> [w370]
    tunnel: w22 -> [w369]
    tunnel: w21 -> [w368]
    tunnel: w19 -> [_]
    tunnel: w3 -> [w367]
    stop <- FALSE stop-if-true
    n190 = event shown="[15] \"总氮稀释倍数\": 值改变" {
      selector: _ -> [_ _ _ _ _ _ _ _ _ _ _ _ _ _ _ _]
      dyn-events: _ -> [_ _ _ _ _ _ _ _ _ _ _ _ _ _ _ _]
      timeout: _ -> [_ _ _ _ _ _ _ _ _ _ _ _ _ _ _ _]
      tunnel: w374 -> [_ w378 _ w389 w391 _ _ _ _ _ _ _ _ _ _ _]
      tunnel: w373 -> [_ _ _ _ _ _ _ _ _ w444 _ w464 w473 _ _ _]
      tunnel: w372 -> [_ _ _ _ _ _ _ _ _ w442 _ w462 w475 w483 w490 _]
      tunnel: w371 -> [_ _ _ _ _ _ _ _ _ w443 _ w463 w474 _ _ _]
      tunnel: w370 -> [_ _ _ _ _ _ _ _ _ w438 _ _ _ _ _ _]
      tunnel: w369 -> [_ _ _ _ _ _ _ _ _ _ _ w458 _ _ _ _]
      tunnel: w368 -> [_ _ _ _ _ _ _ _ _ _ _ _ _ w481 _ _]
      tunnel: w367 -> [_ _ _ _ _ _ _ _ _ _ _ _ _ _ _ _]
      event Timeout {
        n191 = event-data() -> ()  [unwired: 1 in, 3 out]
      }
      event "手动启动": Value Change {
        n192 = event-data() -> ()  [unwired: 1 in, 6 out]
        n193 = call "总磷氨氮启动参数对话框.vi"() -> ("确认"=w376:bool, "元素"=w377:cluster{"命令":string, "data":variant})  [unwired: 10 in]
        n194 = case shown="真" w376 {
          tunnel: w378 -> [_ w380]
          tunnel: w377 -> [_ w379]
          frame False {
          }
          frame True {
            n195 = Enqueue Element(queue=w380, element=w379) -> ()  [unwired: 2 in, 3 out]
          }
        }
      }
      event "定时启动": Mouse Down {
        n196 = event-data() -> ()  [unwired: 1 in, 6 out]
        n197 = call "定时启动对话框.vi"() -> ("设置值"=→"设置值":dbl, "确定输出"=→"定时启动":bool)  [unwired: 10 in]
      }
      event "单步测试": Value Change {
        w384 = u16 1 items=["总磷"=1, "氨氮"=3] ("站号")
        n198 = event-data() -> ()  [unwired: 1 in, 6 out]
        n199 = Bundle("站号"=w384, "总磷氨氮调试"="总磷氨氮调试") -> (w383:cluster{"站号":u16, "总磷氨氮调试":u16[]})  [unwired: 1 in]
        n200 = Bundle By Name(cluster=cluster{"命令":string, "data":variant} {"命令"="", "data"=variant} ("元素"), "命令"="debug", "data"=w383) -> (w386:cluster{"命令":string, "data":variant})
        n201 = Enqueue Element(queue=w389, element=w386) -> ()  [unwired: 2 in, 3 out]
      }
      event "停止": Value Change {
        n202 = event-data() -> ()  [unwired: 1 in, 6 out]
        n203 = Enqueue Element(queue=w391, element=cluster{"命令":string, "data":variant} {"命令"="启动", "data"=variant(cluster{"站号":u16, "控制命令输出":u16[]} {"站号"=1, "控制命令输出"=[2816]})} ("元素")) -> ()  [unwired: 2 in, 3 out]
      }
      event "设置": Value Change {
        n204 = event-data() -> ()  [unwired: 1 in, 6 out]
        n205 = property on="窗格" class="Pane"("Origin"=T5 {"Horizontal"=0, "Vertical"=628} ("原点")) -> ()  [unwired: 2 in, 2 out]
      }
      event "返回": Value Change {
        n206 = event-data() -> ()  [unwired: 1 in, 6 out]
        n207 = property on="窗格" class="Pane"("Origin"=T5 {"Horizontal"=0, "Vertical"=0} ("原点")) -> ()  [unwired: 2 in, 2 out]
      }
      event "标液浓度1", "测量吸光度1", "测量吸光度2", "标液浓度2", "测量吸光度3", "标液浓度3", "测量吸光度4", "标液浓度4", "测量吸光度5", "标液浓度5", "样品1启用", "样品3启用", "样品4启用", "样品5启用", "样品2启用", "模型", "method", "样品1 F0", "样品1 F1", "样品2 F1", "样品2 F0", "样品3 F1", "样品4 F0", "样品4 F1", "样品5 F1", "样品5 F0", "精度": Value Change {
        n208 = event-data() -> ()  [unwired: 1 in, 6 out]
        n209 = formula code="E=log(F0/F1);"("F0"="样品1 F0", "F1"="样品1 F1") -> ("E"=w415:dbl)
        "测量吸光度1" <- w415
        n210 = formula code="E=log(F0/F1);"("F0"="样品2 F0", "F1"="样品2 F1") -> ("E"=w412:dbl)
        "测量吸光度2" <- w412
        n211 = formula code="E=log(F0/F1);"("F0"="样品3 F0", "F1"="样品3 F1") -> ("E"=w409:dbl)
        "测量吸光度3" <- w409
        n212 = formula code="E=log(F0/F1);"("F0"="样品4 F0", "F1"="样品4 F1") -> ("E"=w406:dbl)
        "测量吸光度4" <- w406
        n213 = formula code="E=log(F0/F1);"("F0"="样品5 F0", "F1"="样品5 F1") -> ("E"=w403:dbl)
        "测量吸光度5" <- w403
        n214 = Replace Array Subset(array=dbl[] [0.0, 0.0, 0.0, 0.0, 0.0] ("数组"), new element #1="标液浓度1", new element #2="标液浓度2", new element #3="标液浓度3", new element #4="标液浓度4", new element #5="标液浓度5") -> (w400:dbl[])  [unwired: 5 in]
        n215 = Replace Array Subset(array=dbl[] [0.0, 0.0, 0.0, 0.0, 0.0] ("数组"), new element #1=w415, new element #2=w412, new element #3=w409, new element #4=w406, new element #5=w403) -> (w399:dbl[])  [unwired: 5 in]
        n216 = Replace Array Subset(array=bool[] [FALSE, FALSE, FALSE, FALSE, FALSE] ("数组"), new element #1="样品1启用", new element #2="样品2启用", new element #3="样品3启用", new element #4="样品4启用", new element #5="样品5启用") -> (w398:bool[])  [unwired: 5 in]
        n217 = call "线性公式.vi"("精度"="精度", "模型"="模型", "method"="method", "启用"=w398, "监测浓度"=w399, "标液浓度"=w400) -> ("XY图"=→"XY图":cluster{"X Values":dbl[], "Y Values":dbl[]}[], "r^2"=→"r^2":dbl, "拟合方程"=→"拟合公式":string)  [unwired: 3 in]
      }
      event "标液浓度1", "标液浓度2", "标液浓度3", "标液浓度4", "标液浓度5", "样品1 F0", "样品1 F1", "样品2 F1", "样品2 F0", "样品3 F1", "样品3 F0", "样品4 F0", "样品4 F1", "样品5 F0", "样品5 F1", "精度", "公式.X^2", "公式.X", "公式.b", "量程切换阈值.阈值", "量程切换阈值.标液浓度", "备用系数.量程上限", "备用系数.量程下限", "备用系数.检出限", "备用系数.精度", "总氮稀释倍数": Mouse Down {
        n218 = event-data() -> ("CtlRef"=w434:refnum<vi>)  [unwired: 1 in, 5 out]
        n219 = property class="DigNum (严格)"(reference=w434) -> (reference out=w432:refnum<vi>, "Value"=w433:dbl)  [unwired: 1 in, 1 out]
        n220 = call "数字键盘.vi"("OldNumber"=w433) -> ("NewNumber"=w431:sgl)
        n221 = property class="DigNum (严格)"(reference=w432, "Val(Sgnl)"=w431) -> ()  [unwired: 1 in, 2 out]
      }
      event "读公式": Value Change {
        n222 = event-data() -> ()  [unwired: 1 in, 6 out]
        n223 = property class="Enum (严格)"(reference=w442) -> ("Value"=w441:enum16{"总磷", "总氮"})  [unwired: 1 in, 2 out]
        n224 = property class="Enum (严格)"(reference=w443) -> ("Value"=w440:enum16{"水样测量", "空白核查", "跨度核查", "标样核查", "加标回收"})  [unwired: 1 in, 2 out]
        n225 = property class="Enum (严格)"(reference=w444) -> ("Value"=w439:enum16{"低量程", "高量程"})  [unwired: 1 in, 2 out]
        n226 = call "总磷氨氮公式读取.vi"("量程"=w439, "测量模式"=w440, "测量参数"=w441) -> ("error out"=w436:errorcluster, "公式"=w437:cluster{"X^2":dbl, "X":dbl, "b":dbl})  [unwired: 7 in]
        n227 = property class="Clust (严格)"(reference=w438, "Value"=w437) -> ()  [unwired: 1 in, 2 out]
        n228 = case shown="错误" w436 {
          tunnel: ["读取成功" ("消息") "读取失败" ("消息")] -> w435
          frame No Error {
          }
          frame Error {
          }
        }
        n229 = One Button Dialog(message=w435) -> ()  [unwired: 1 in, 1 out]
      }
      event "写公式": Value Change {
        n230 = event-data() -> ()  [unwired: 1 in, 6 out]
        n231 = call "总磷氨氮公式写入.vi"("公式"="公式", "量程"="量程下拉列表", "测量模式"="测量模式下拉列表", "测量参数"="参数下拉列表") -> ("error out"=w449:errorcluster)  [unwired: 7 in]
        n232 = case shown="无错误" w449 {
          tunnel: ["写入成功" ("消息") "写入失败" ("消息")] -> w450
          frame No Error {
          }
          frame Error {
          }
        }
        n233 = One Button Dialog(message=w450) -> ()  [unwired: 1 in, 1 out]
      }
      event "量程切换阈值读取": Value Change {
        n234 = event-data() -> ()  [unwired: 1 in, 6 out]
        n235 = property class="Enum (严格)"(reference=w462) -> ("Value"=w461:enum16{"总磷", "总氮"})  [unwired: 1 in, 2 out]
        n236 = property class="Enum (严格)"(reference=w463) -> ("Value"=w460:enum16{"水样测量", "空白核查", "跨度核查", "标样核查", "加标回收"})  [unwired: 1 in, 2 out]
        n237 = property class="Enum (严格)"(reference=w464) -> ("Value"=w459:enum16{"低量程", "高量程"})  [unwired: 1 in, 2 out]
        n238 = call "总磷氨氮量程读取.vi"("量程"=w459, "测量模式"=w460, "测量参数"=w461) -> ("error out"=w455:errorcluster, "量程切换阈值"=w457:cluster{"阈值":dbl, "标液浓度":dbl})  [unwired: 7 in]
        n239 = property class="Clust (严格)"(reference=w458, "Value"=w457) -> ()  [unwired: 1 in, 2 out]
        n240 = case shown="错误" w455 {
          tunnel: ["读取成功" ("消息") "读取失败" ("消息")] -> w456
          frame No Error {
          }
          frame Error {
          }
        }
        n241 = One Button Dialog(message=w456) -> ()  [unwired: 1 in, 1 out]
      }
      event "量程切换阈值写入": Value Change {
        n242 = event-data() -> ()  [unwired: 1 in, 6 out]
        n243 = property class="Enum (严格)"(reference=w475) -> ("Value"=w472:enum16{"总磷", "总氮"})  [unwired: 1 in, 2 out]
        n244 = property class="Enum (严格)"(reference=w474) -> ("Value"=w471:enum16{"水样测量", "空白核查", "跨度核查", "标样核查", "加标回收"})  [unwired: 1 in, 2 out]
        n245 = property class="Enum (严格)"(reference=w473) -> ("Value"=w470:enum16{"低量程", "高量程"})  [unwired: 1 in, 2 out]
        n246 = call "总磷氨氮量程写入.vi"("量程切换阈值"="量程切换阈值", "量程"=w470, "测量模式"=w471, "测量参数"=w472) -> ("error out"=w467:errorcluster)  [unwired: 7 in]
        n247 = case shown="无错误" w467 {
          tunnel: ["写入成功" ("消息") "写入失败" ("消息")] -> w468
          frame No Error {
          }
          frame Error {
          }
        }
        n248 = One Button Dialog(message=w468) -> ()  [unwired: 1 in, 1 out]
      }
      event "备用系数读取": Value Change {
        n249 = event-data() -> ()  [unwired: 1 in, 6 out]
        n250 = property class="Enum (严格)"(reference=w483) -> ("Value"=w482:enum16{"总磷", "总氮"})  [unwired: 1 in, 2 out]
        n251 = call "总磷氨氮备用系数读取.vi"("测量参数"=w482) -> ("error out"=w478:errorcluster, "备用系数"=w480:T1)  [unwired: 9 in]
        n252 = property class="Clust (严格)"(reference=w481, "Value"=w480) -> ()  [unwired: 1 in, 2 out]
        n253 = case shown="错误" w478 {
          tunnel: ["读取成功" ("消息") "读取失败" ("消息")] -> w479
          frame No Error {
          }
          frame Error {
          }
        }
        n254 = One Button Dialog(message=w479) -> ()  [unwired: 1 in, 1 out]
      }
      event "备用系数写入": Value Change {
        n255 = event-data() -> ()  [unwired: 1 in, 6 out]
        n256 = property class="Enum (严格)"(reference=w490) -> ("Value"=w489:enum16{"总磷", "总氮"})  [unwired: 1 in, 2 out]
        n257 = call "总磷氨氮备用系数写入.vi"("备用系数"="备用系数", "测量参数"=w489) -> ("error out"=w486:errorcluster)  [unwired: 9 in]
        n258 = case shown="无错误" w486 {
          tunnel: ["写入成功" ("消息") "写入失败" ("消息")] -> w487
          frame No Error {
          }
          frame Error {
          }
        }
        n259 = One Button Dialog(message=w487) -> ()  [unwired: 1 in, 1 out]
      }
      event "总氮稀释倍数": Value Change {
        n260 = event-data() -> ()  [unwired: 1 in, 6 out]
        n261 = call <vilib>:"Application Directory.vi"() -> ("Application Directory"=w500:path)
        n262 = Build Path(base path=w500, name or relative path="data\\Set.ini" ("名称或相对路径")) -> (appended path=w502:path)
        n263 = local read "总氮稀释倍数"() -> (w495:dbl)
        n264 = call <vilib>:"Open Config Data.vi"("configuration file path"=w502) -> ("error out"=w497:errorcluster, "refnum"=w499:T16)  [unwired: 8 in, 1 out]
        n265 = global write "VAR总磷氨氮全局变量.vi" "总氮稀释倍数"(w495) -> ()
        n266 = call-poly <vilib>:"Write Key.vi"("section"="总磷总氮", "error in (no error)"=w497, "value"=w495, "key"="总氮稀释倍数" ("section"), "refnum"=w499) -> ("error out"=w496:errorcluster, "refnum out"=w498:T16)  [unwired: 4 in, 1 out]
        n267 = call <vilib>:"Close Config Data.vi"("error in (no error)"=w496, "refnum"=w498) -> ()  [unwired: 8 in, 2 out]
      }
    }
  }
  n268 = while {
    tunnel: w46 -> [w519]
    tunnel: w47 -> [_]
    shift-right: [w511] -> _
    shift-left: enum16{"总磷", "总氮"}."总磷" ("枚举") -> [w513]
    stop <- FALSE stop-if-true
    # "试剂填充 172 \n管路清洗108\n氨氮92\n总磷131\n总磷海水147\n总氮76\n总氮海水92"
    n269 = case shown="\"总氮\", 默认" w513 {
      selector: w513 -> [w528 w530]
      tunnel: [w529 w531] -> w514
      tunnel: [w528 w530] -> w512
      frame "总氮", Default {
        w529 = u16 2 items=["总磷"=1, "总氮"=2] ("站号")
      }
      frame "总磷" {
        w531 = u16 1 items=["总磷"=1, "氨氮"=3] ("站号")
      }
    }
    n270 = Wait (ms)(milliseconds to wait=u32 1000 ("等待时间（毫秒）")) -> ()  [unwired: 1 out]
    n271 = Bundle By Name(cluster=cluster{"命令":string, "data":variant} {"命令"="", "data"=variant} ("元素"), "命令"="读状态告警区", "data"=w514) -> (w521:cluster{"命令":string, "data":variant})
    n272 = global read "VAR总磷氨氮全局变量.vi" "状态告警区"() -> (w503:T3)
    n273 = Unbundle By Name(w503) -> ("系统时间"=w510:timestamp)
    n274 = Enqueue Element(queue=w519, element=w521) -> (queue out=w515:refnum<queue>)  [unwired: 2 in, 2 out]
    n275 = Get Date/Time In Seconds() -> (seconds since 1Jan1904=w509:timestamp)
    n276 = Subtract(x=w509, y=w510) -> (x-y=w508:dbl)
    n277 = Bundle By Name(cluster=cluster{"命令":string, "data":variant} {"命令"="", "data"=variant} ("元素"), "命令"="读测量数据区", "data"=w514) -> (w517:cluster{"命令":string, "data":variant})
    n278 = Absolute Value(x=w508) -> (abs(x)=w507:dbl)
    n279 = Enqueue Element(queue=w515, element=w517) -> (queue out=w504:refnum<queue>)  [unwired: 2 in, 2 out]
    n280 = Greater Or Equal?(x=w507, y=120.0) -> (x >= y?=w505:bool)
    n281 = case shown="真" w505 {
      tunnel: w504 -> [_ w526]
      frame False {
      }
      frame True {
        n282 = call "总磷氨氮启动命令.vi"("参数"=T18 {"站号"=3, "量程切换"=enum."AUTO", "控制命令"=enum."校时", "模式设置"=enum."待机", "测量间隔"=0}) -> ("启动命令"=w525:cluster{"命令":string, "data":variant})  [unwired: 10 in]
        n283 = Enqueue Element(queue=w526, element=w525) -> ()  [unwired: 2 in, 3 out]
      }
    }
    n284 = Increment(x=w512) -> (x+1=w511:enum16{"总磷", "总氮"})
  }
